vi "Array to XY (N Ch).vi"(8 "channel names":string[](array[string]), 10 "Y data":dbl[](array[numeric]), 11 "X data":dbl[](array[numeric])) -> (3 "XY plots":cluster{"X data":dbl[], "Y data":dbl[]}[](array[cluster]))   [LabVIEW 2023]
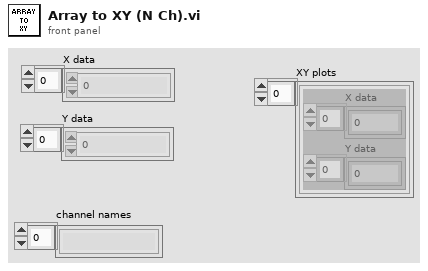
[diagram p1: front panel]
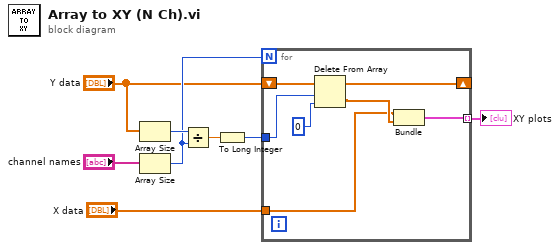
[diagram p0: block diagram]
diagram:
  n1 = Array Size(array="Y data") -> (size(s)=w8:i32)
  n2 = Array Size(array="channel names") -> (size(s)=w7:i32)
  n3 = Divide(x=w8, y=w7) -> (x/y=w5:dbl)
  n4 = To Long Integer(number=w5) -> (32bit integer=w4:i32)
  n5 = for {
    N: w7 -> [_]
    shift-right: [w14] -> _
    shift-left: "Y data" -> [w15]
    tunnel: w4 -> [w12]
    tunnel: "X data" -> [w10]
    tunnel: [w9] -> w1 mode=indexing
    n6 = Delete From Array(array=w15, length=w12, index=0) -> (deleted portion=w11:dbl[], array with subset deleted=w14:dbl[])
    n7 = Bundle("X data"=w10, "Y data"=w11) -> (w9:cluster{"X data":dbl[], "Y data":dbl[]})  [unwired: 1 in]
  }
  "XY plots" <- w1
